vi "tcsOfc_waitForCompletion_readWfsFile.vi"(8 "error in (no error)":errorcluster, 11 "waitComplete_Ctl":cluster{"cmdSeqNum":i32, "timeout":u32}) -> (0 "error out":errorcluster, 2 "function return":i32, 3 "waitComplete_Ctl out":cluster{"cmdSeqNum":i32, "timeout":u32})   [LabVIEW 2016, in "SALLV_tcsOfc.lvlib"]
doc: "int tcsOfc_shm_waitForCompletion_readWfsFileLV(tcsOfc_waitCompleteLV *waitComplete_Ctl);"
uses:
  SALLV_tcsOfc.lvlib
  SALLV_tcsOfc.so
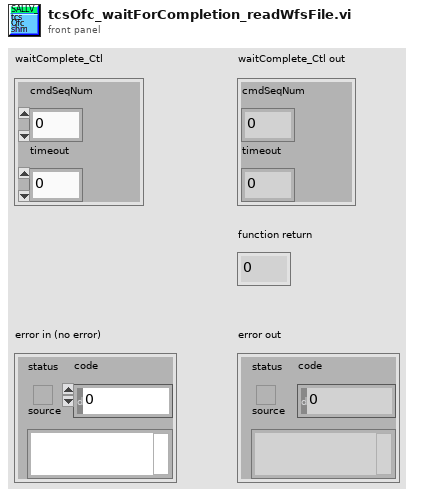
[diagram p1: front panel]
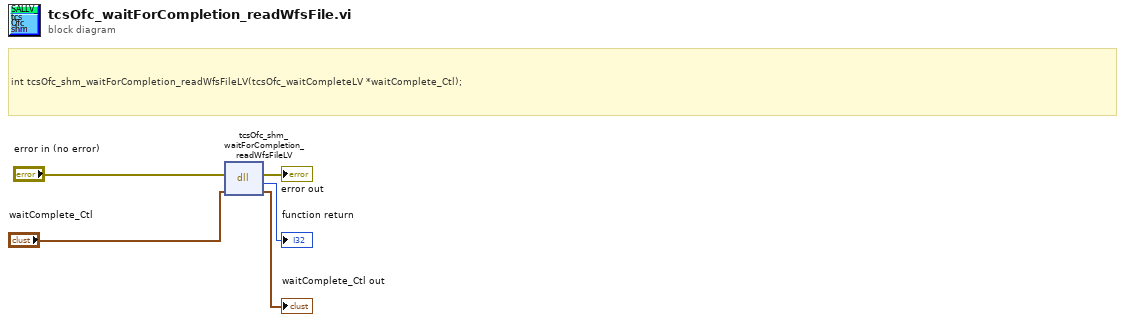
[diagram p0: block diagram]
diagram:
  # "int tcsOfc_shm_waitForCompletion_readWfsFileLV(tcsOfc_waitCompleteLV *waitComplete_Ctl);"
  n1 = dll-call lib="home/ttsai/Documents/salAPI/SALLV_tcsOfc/SALLV_tcsOfc.*" fn="tcsOfc_shm_waitForCompletion_readWfsFileLV"(error in="error in (no error)", "waitComplete_Ctl"="waitComplete_Ctl") -> (error out=→"error out":errorcluster, →"function return":i32, "waitComplete_Ctl"=→"waitComplete_Ctl out":cluster{"cmdSeqNum":i32, "timeout":u32})  [unwired: 2 in, 1 out]
